vi "Configure Clock Recovery Method JTF.vi"(0 "VISA resource name":refnum<visa-resource-name>, 1 "Recovery Method (0: First Order PLL)":i32(ring) items=["First Order PLL", "Second Order PLL", "Equalized First Order PLL", "Equalized Second Order PLL", "Explicit First Order PLL", "Explicit Second Order PLL"], 2 "Data Rate (0)":dbl, 3 "Peaking / Damping Factor (0)":dbl, 5 "Setting Terms (0: JTF)":i32(ring) items=["JTF", "OJTF"], 7 "Loop Bandwidth (0)":dbl, 9 "Clock Edge (0: Rising)":i32(ring) items=["Rising", "Falling", "Both"], 11 "error in (no error)":errorcluster, 12 "Multiplication Factor (0)":i32, 13 "Clock Frequency (0)":dbl, 14 "Measurement Source (1: Channel 1)":i32(ring)=1 items=["Channel 1"=1, "Channel 2"=2, "Channel 3"=3, "Channel 4"=4, "Function 1"=5, "Function 2"=6, "Function 3"=7, "Function 4"=8, "Memory 1"=9, "Memory 2"=10, "Memory 3"=11, "Memory 4"=12]) -> (4 "VISA resource name out":refnum<visa-resource-name>, 15 "error out":errorcluster)   [LabVIEW 2013, in "Agilent 90000 Series.lvlib"]
doc: "Configures the clock recovery PLL's response."
uses:
  Agilent 90000 Series.lvlib
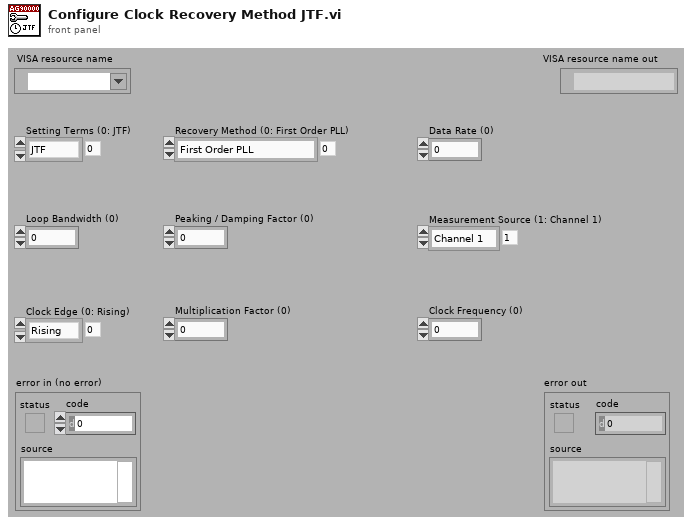
[diagram p1: front panel]
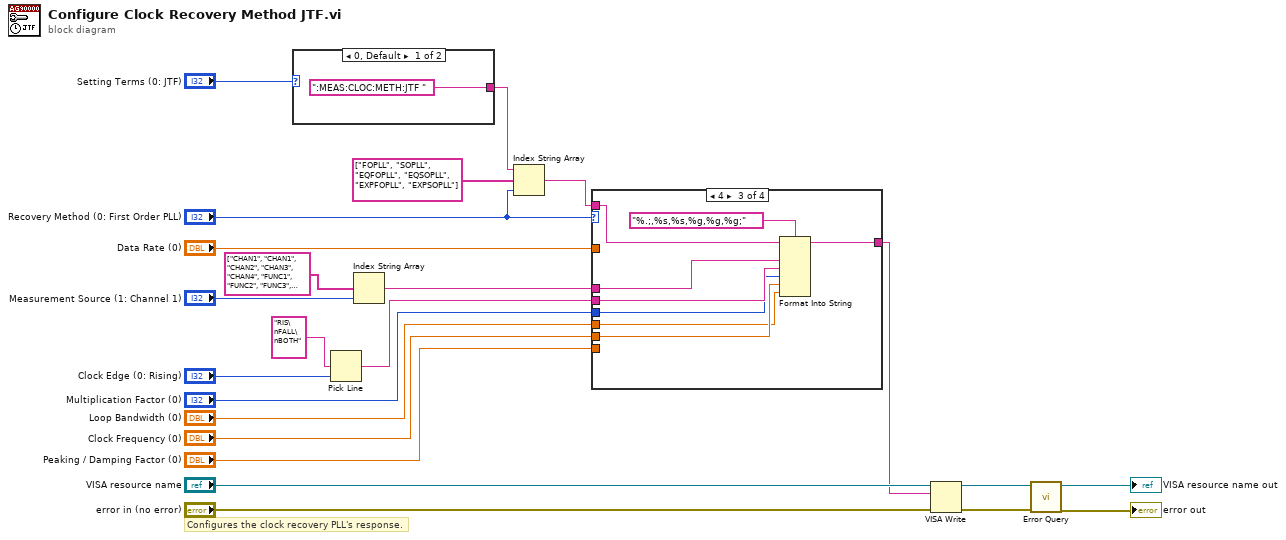
[diagram p0: block diagram]
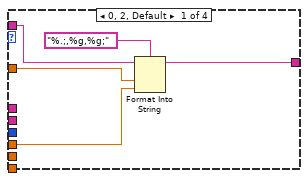
[diagram p2: hidden frame]
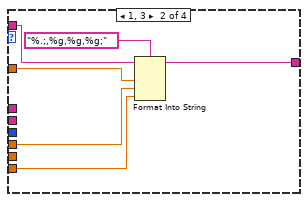
[diagram p3: hidden frame]
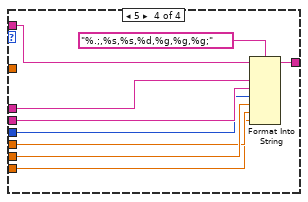
[diagram p4: hidden frame]
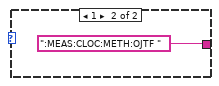
[diagram p5: hidden frame]
diagram:
  # "Configures the clock recovery PLL's response."
  n1 = case shown="0, Default" "Setting Terms (0: JTF)" {
    tunnel: [":MEAS:CLOC:METH:JTF " ":MEAS:CLOC:METH:OJTF "] -> w13
    frame 0, Default {
    }
    frame 1 {
    }
  }
  n2 = Pick Line(multi-line string="RIS\nFALL\nBOTH", line index="Clock Edge (0: Rising)") -> (output string=w4:string)  [unwired: 1 out]
  n3 = Index String Array(1:"Measurement Source (1: Channel 1)", 2:string[] ["CHAN1", "CHAN1", "CHAN2", "CHAN3", "CHAN4", "FUNC1", "FUNC2", "FUNC3", "FUNC4", "WMEM1", "WMEM2", "WMEM3", "WMEM4"] ("subarray 2")) -> (0:w5:string)  [unwired: 1 out]
  n4 = Index String Array(1:"Recovery Method (0: First Order PLL)", 2:string[] ["FOPLL", "SOPLL", "EQFOPLL", "EQSOPLL", "EXPFOPLL", "EXPSOPLL"], 3:w13) -> (0:w9:string)
  n5 = case shown="4" "Recovery Method (0: First Order PLL)" {
    tunnel: "Data Rate (0)" -> [w29 w35 _ _]
    tunnel: "Loop Bandwidth (0)" -> [w28 w34 w39 w48]
    tunnel: w9 -> [w27 w32 w38 w46]
    tunnel: "Peaking / Damping Factor (0)" -> [_ w33 _ w47]
    tunnel: w5 -> [_ _ w43 w52]
    tunnel: w4 -> [_ _ w42 w51]
    tunnel: "Multiplication Factor (0)" -> [_ _ w41 w50]
    tunnel: "Clock Frequency (0)" -> [_ _ w40 w49]
    tunnel: [w26 w31 w37 w45] -> w1
    frame 0, 2, Default {
      n6 = Format Into String(format string="%.;,%g,%g;", initial string=w27, w29, w28) -> (resulting string=w26:string)  [unwired: 1 in, 1 out]
    }
    frame 1, 3 {
      n7 = Format Into String(format string="%.;,%g,%g,%g;", initial string=w32, w35, w34, w33) -> (resulting string=w31:string)  [unwired: 1 in, 1 out]
    }
    frame 4 {
      n8 = Format Into String(format string="%.;,%s,%s,%g,%g,%g;", initial string=w38, w43, w42, w41, w40, w39) -> (resulting string=w37:string)  [unwired: 1 in, 1 out]
    }
    frame 5 {
      n9 = Format Into String(format string="%.;,%s,%s,%d,%g,%g,%g;", initial string=w46, w52, w51, w50, w49, w48, w47) -> (resulting string=w45:string)  [unwired: 1 in, 1 out]
    }
  }
  n10 = VISA Write(VISA resource name="VISA resource name", write buffer=w1, error in (no error)="error in (no error)") -> (VISA resource name out=w19:refnum<visa-resource-name>, error out=w18:errorcluster)  [unwired: 1 out]
  n11 = call "Error Query.vi"("error in (no error)"=w18, "VISA resource name"=w19) -> ("error out"=→"error out":errorcluster, "VISA resource name out"=→"VISA resource name out":refnum<visa-resource-name>)  [unwired: 8 out]
